vi "TrayROIArr.vi"() -> ()   [LabVIEW 2019]
uses:
  <vilib>/Utility/miscctls.llb/LVRowAndColumnTypeDef.ctl
  <vilib>/Utility/miscctls.llb/LVPointTypeDef.ctl
  <vilib>/vision/Image Controls.llb/IMAQ Image.ctl
  <vilib>/vision/Pattern Matching.llb/IMAQ Pattern Match Advanced Options.ctl
  Auto Inspection Tray Map Name.ctl
  54da9b37-9451-4d09-bda1-2468331c8fce.vi
  3a246969-8a69-47b9-98d6-f50759c243ea.vi
  cc50742a-40e5-4032-86be-5ab09aa8e016.vi
  36dc4686-89ba-4588-a2d3-35b5f35309b2.vi
  d60a80a8-80a4-4e46-9028-f9893c6610f3.vi
  <vilib>/JDP Science/JSONtext/Variant to JSON Text.vi
  <vilib>/JDP Science/JSONtext/JSON text to Variant.vi
  LLB/Commonly VI.lvlib
  <vilib>/vision/NI_Vision_Development_Module.lvlib
  LLB/Commonly VI/Main Glb.vi
panel:
  out "Matches (pixel)":T1(array[cluster]) {"Bounding Box"."y" format="%.2f"; "Bounding Box"."x" format="%.2f"; "Score" format="%.2f"; "Scale" format="%.2f"; "Angle" format="%.2f"; "Position"."y" format="%.2f"; "Position"."x" format="%.2f"}
  in  "ImgCut":bool
  in  "Project":string
  in  "LSCopyFrom":u16(ring) items=["Area1", "Area2"]
  in  "LSXNum":i32 caption="XNum"
  in  "LSYNum":i32 caption="YNum"
  in  "LSXDist":i32 caption="XDist"
  in  "LSYDist":i32 caption="YDist"
  out "LSTotalTrayArea":string[][](table) caption="料盤區塊對應"
  in  "LSAnalysisProject":u16(ring) caption="AnalysisProject" items=["22", "33", "44", "55"]
  in  "AIAnalysisProject":u16(ring) caption="AnalysisProject" items=["22", "33", "44", "55"]
  out "Cell Position":T2
  in  "LSAreaSelect":u16(ring)
  in  "Tab Control":enum32{"LineScan"}(tab)
  in  "Stop Button":bool
  in  "Btn_LSAreaCoordSet":bool
  in  "Save Folder":path
  out "Image":T3(plugin-control)
  in  "Btn_LSAreaDataSet":bool
  out "LS Image":T3(plugin-control)
  in  "Photo":bool
  in  "Btn_LSROITryrun":bool
  in  "Btn_Save":bool
  in  "FolderCut":bool
  in  "Source Folder":path
  in  "定位開啟":bool
  in  "Tab Control 2":enum32{"定位Table", "區域Table"}(tab)
  in  "LSAreaROI 2":i32(listbox) caption="AreaCoordROI"
  in  "LSAreaROI":i32(listbox) caption="AreaROI"
  # "AX     RX個\n\nAY     RY個\n\nN\n\nAY*(N/RX)....."
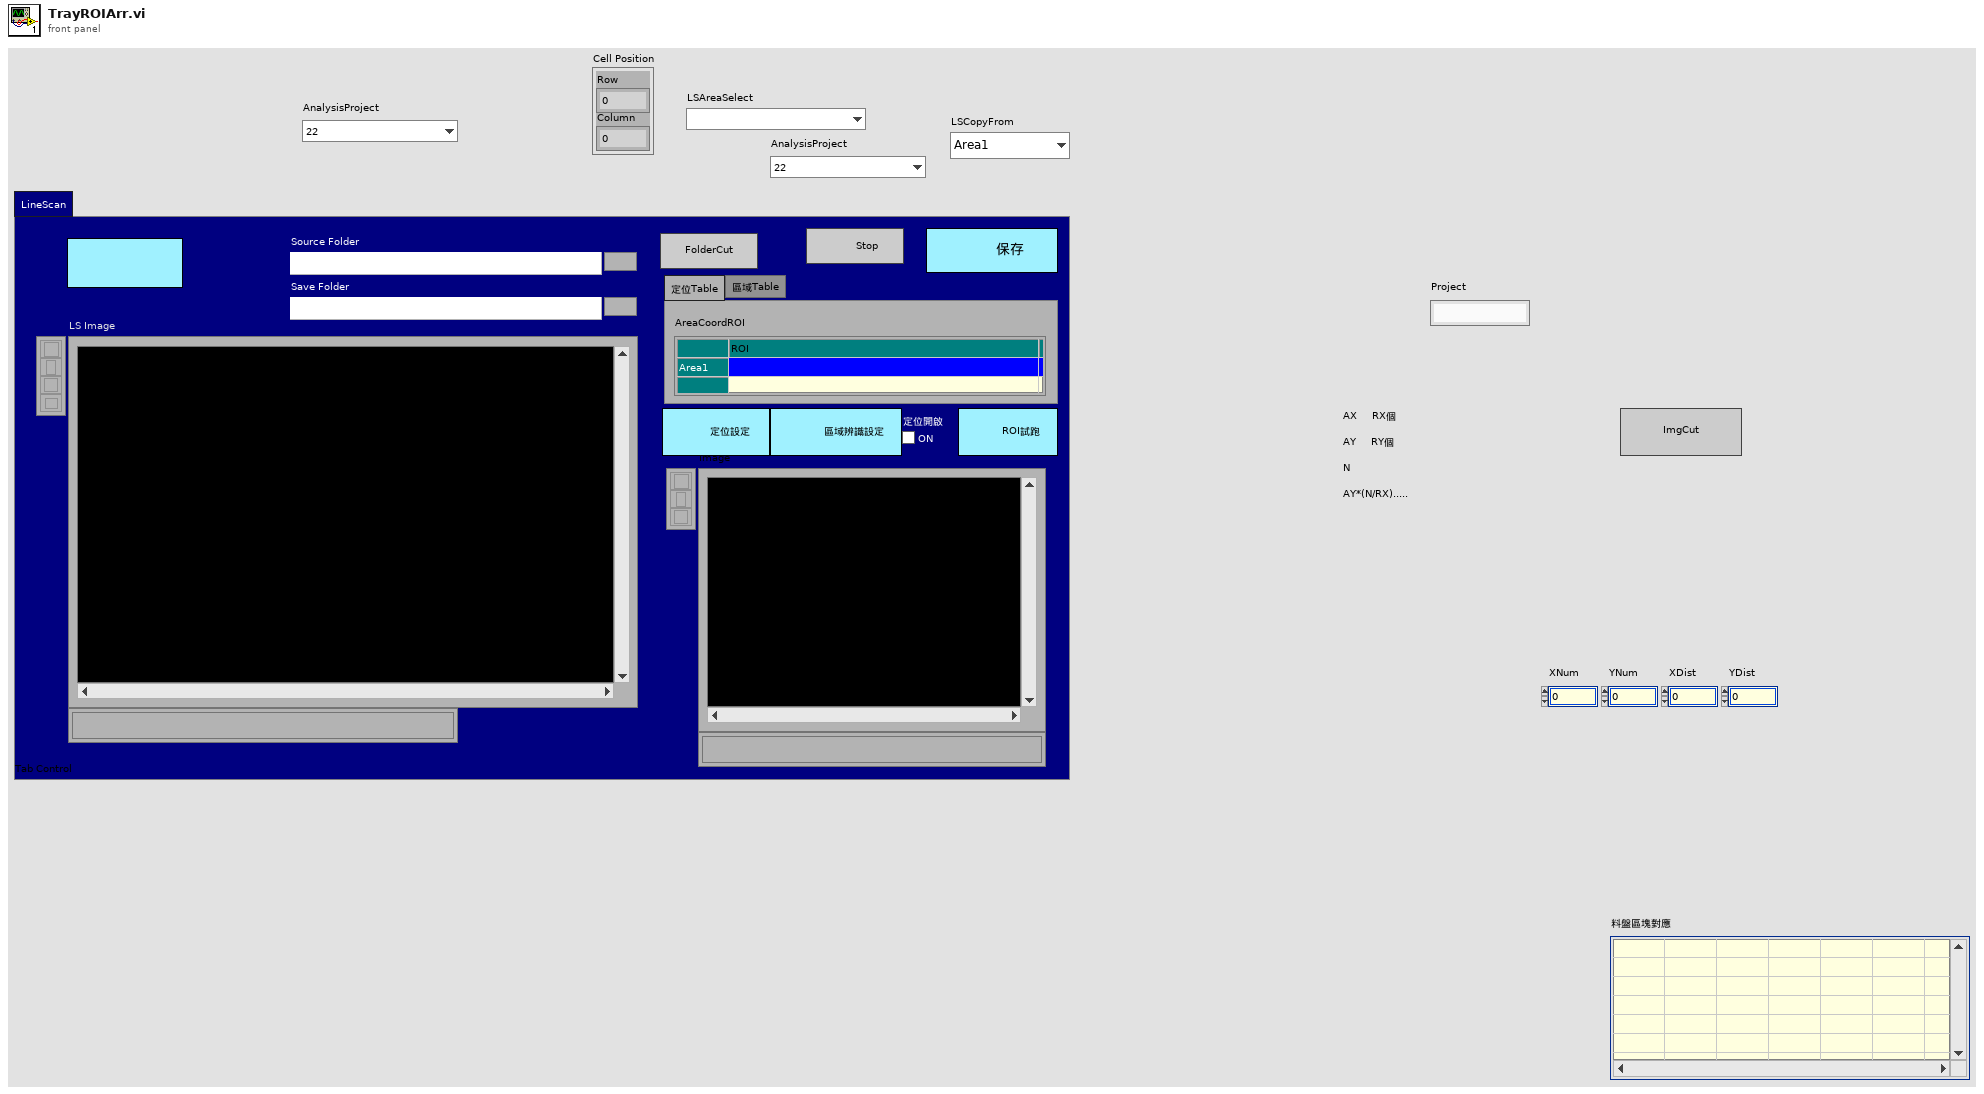
[diagram p1: front panel]
types:
  T1 = cluster{"Position":cluster{"x":sgl, "y":sgl}, "Angle":sgl, "Scale":sgl, "Score":sgl, "Bounding Box":cluster{"x":sgl, "y":sgl}[]}[]
  T2 = typedef "LVRowAndColumnTypeDef.ctl" = cluster{"Row":i32, "Column":i32}
  T3 = typedef "IMAQ Image.ctl" = refnum<image>
  T4 = typedef "LVPointTypeDef.ctl" = cluster{"Horizontal":i16, "Vertical":i16}
  T5 = enum16{"Initial", "Write", "Read", "Save", "Load", "WrteAll"}
  T6 = typedef "IMAQ Pattern Match Advanced Options.ctl" = u16
  T7 = cluster{"Global Rectangle":i32[], "Contours":cluster{"Contour Type":u32, "ROI Type":u32, "Points":i32[]}[]}
  T8 = cluster{"Number of Matches Requested":i32, "Minimum Match Score":sgl, "Angle Ranges":cluster{"Start Angle":sgl, "End Angle":sgl}[]}
  T9 = typedef "Auto Inspection Tray Map Name.ctl" = enum16{"LSTable", "AITable", "LSMap", "AIMap"}
  T10 = typedef "Image Type" = u32
  T11 = typedef "LVPoint32TypeDef.ctl" = cluster{"Horizontal":i32, "Vertical":i32}
  T12 = cluster{"Global Rectangle":i32[], "Contours":cluster{"ID":enum32{"External", "Internal"}, "Type":u32, "Coordinates":i32[]}[]}
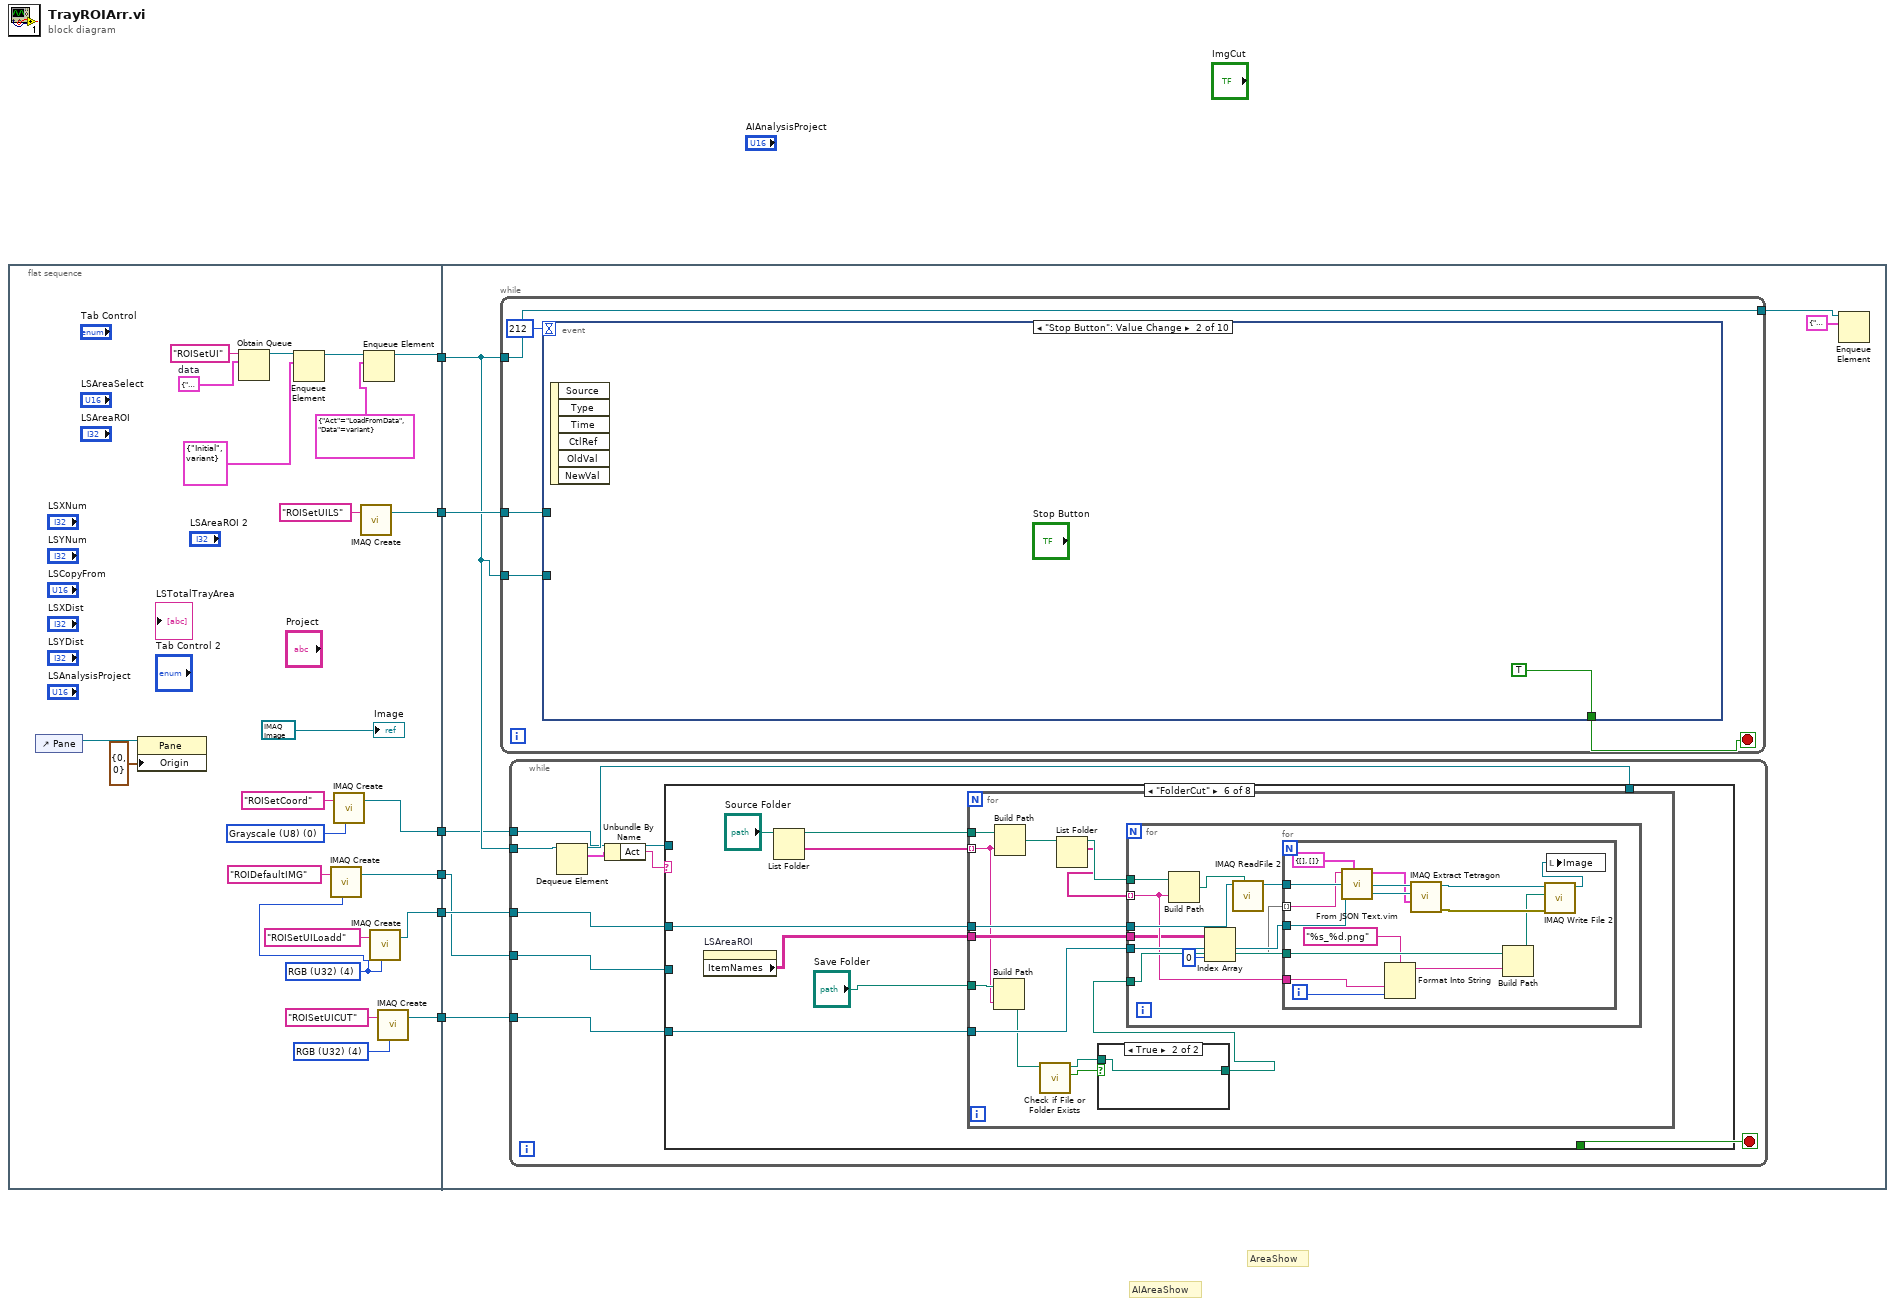
[diagram p0: block diagram]
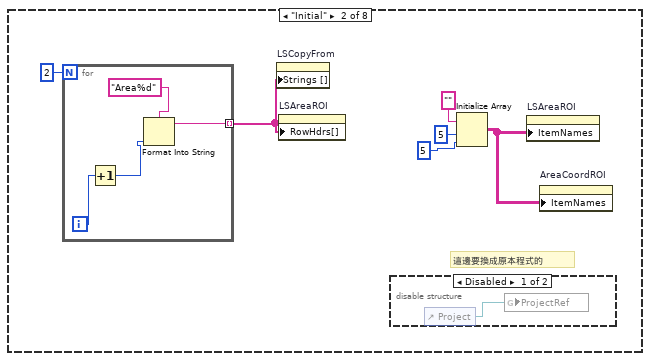
[diagram p3: hidden frame]
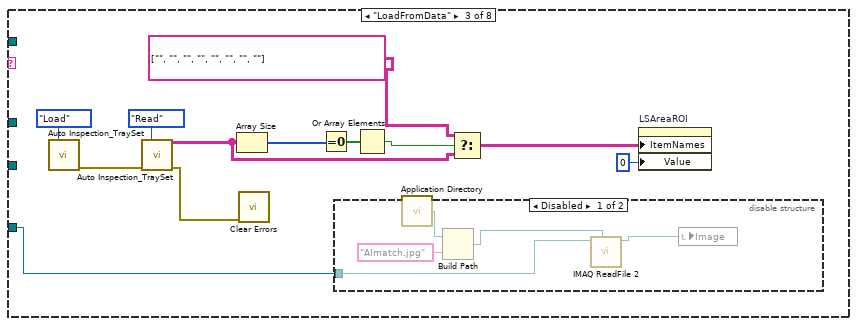
[diagram p5: hidden frame]
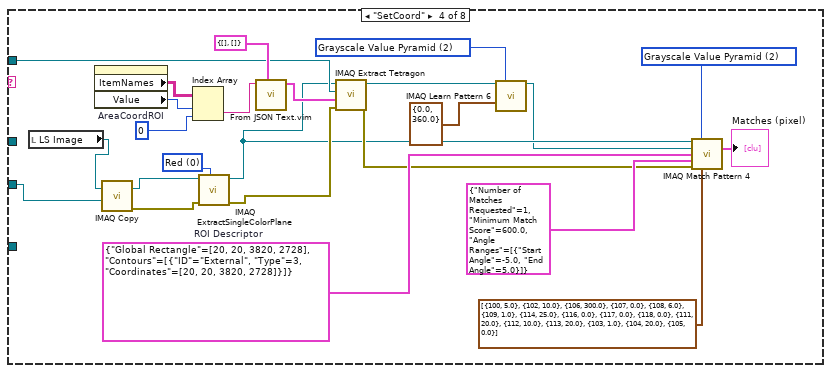
[diagram p7: hidden frame]
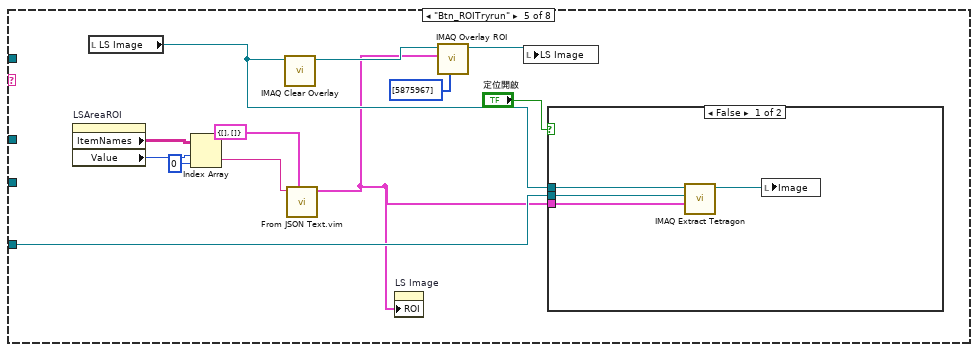
[diagram p8: hidden frame]
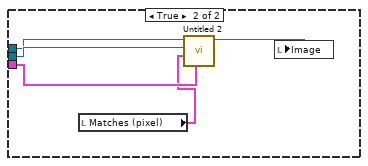
[diagram p9: hidden frame]
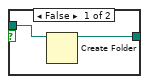
[diagram p10: hidden frame]
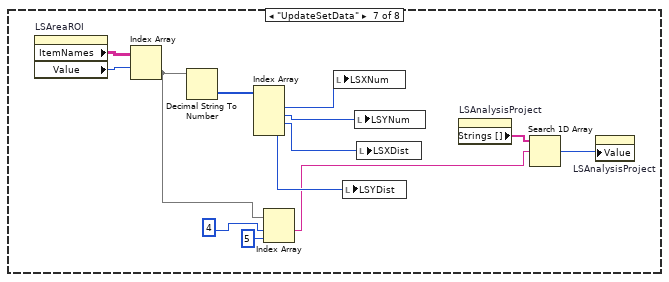
[diagram p11: hidden frame]
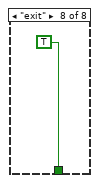
[diagram p12: hidden frame]
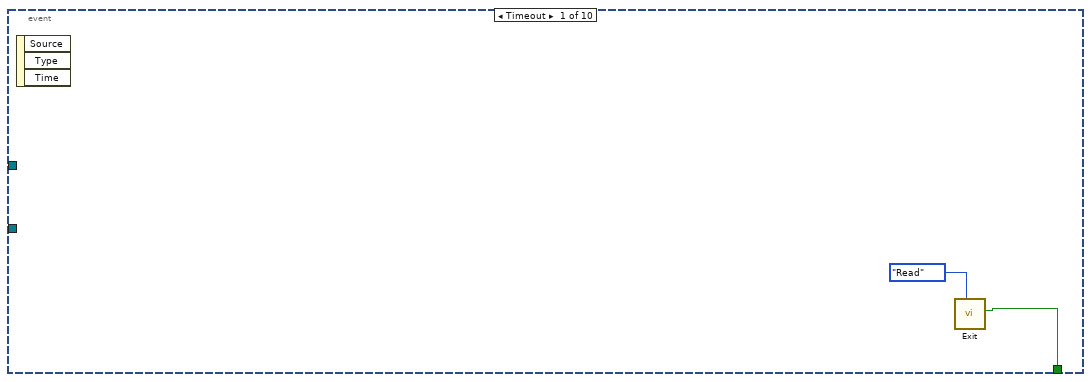
[diagram p13: hidden frame]
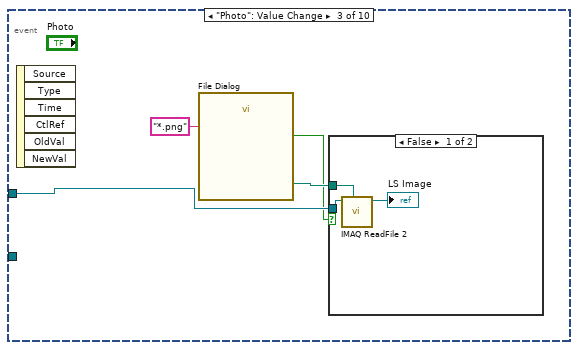
[diagram p14: hidden frame]
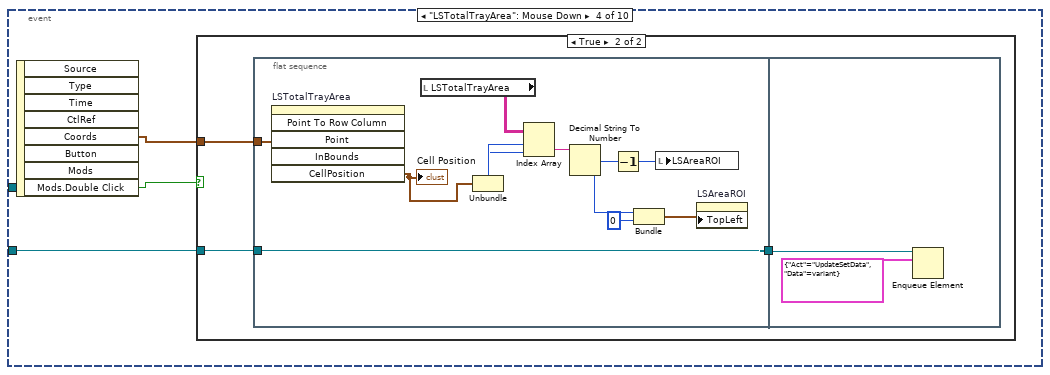
[diagram p16: hidden frame]
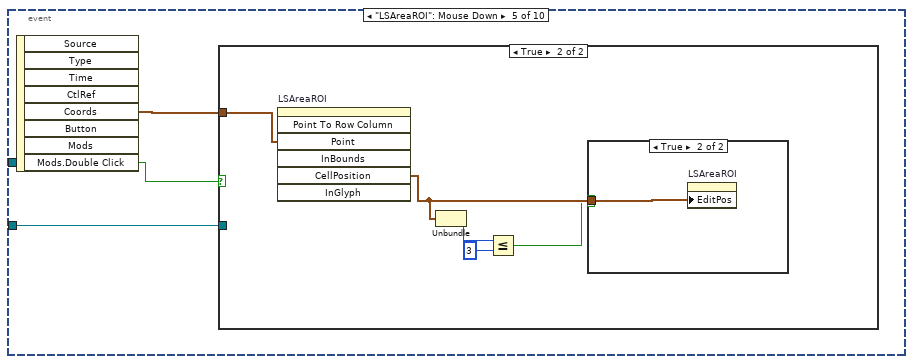
[diagram p18: hidden frame]
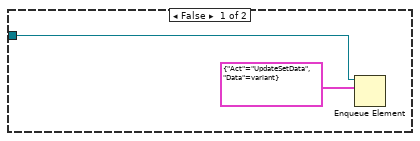
[diagram p19: hidden frame]
diagram:
  # "AreaShow"
  # "AIAreaShow"
  n1 = flat-sequence {
    tunnel: [w21] -> w6
    tunnel: [w24] -> w5
    tunnel: [w16] -> w4
    tunnel: [w14] -> w3
    tunnel: [w12] -> w2
    tunnel: [w10] -> w1
    tunnel: w6 -> [w34]
    tunnel: w5 -> [w35]
    tunnel: w4 -> [w33]
    tunnel: w3 -> [w32]
    tunnel: w2 -> [w31]
    tunnel: w1 -> [w30]
    frame #0 {
      w8 = T10 0 items=["Grayscale (U8)", "Grayscale (I16)", "Grayscale (SGL)", "Complex (CSG)", "RGB (U32)", "HSL (U32)", "RGB (U64)", "Grayscale (U16)"] ("Image Type")
      w9 = T10 4 items=["Grayscale (U8)", "Grayscale (I16)", "Grayscale (SGL)", "Complex (CSG)", "RGB (U32)", "HSL (U32)", "RGB (U64)", "Grayscale (U16)"] ("Image Type")
      w17 = T10 4 items=["Grayscale (U8)", "Grayscale (I16)", "Grayscale (SGL)", "Complex (CSG)", "RGB (U32)", "HSL (U32)", "RGB (U64)", "Grayscale (U16)"] ("Image Type")
      w28 = cluster{"Act":string, "Data":variant} {"Act"="", "Data"=variant}  # data
      n2 = control-ref of="Pane"() -> (w23:refnum<vi>)
      n3 = property class="Pane"(reference=w23, "Origin"=T4 {"Horizontal"=0, "Vertical"=0}) -> ()  [unwired: 1 in, 2 out]
      n4 = Obtain Queue(name (unnamed)="ROISetUI", element data type=w28) -> (queue out=w27:refnum<queue>)  [unwired: 3 in, 2 out]
      n5 = Enqueue Element(queue=w27, element=cluster{"Act":string, "Data":variant} {"Act"="Initial", "Data"=variant}) -> (queue out=w20:refnum<queue>)  [unwired: 2 in, 2 out]
      n6 = call "IMAQ Create"("Image Name"="ROIDefaultIMG", "Image Type"=w9) -> ("New Image"=w10:T3)  [unwired: 3 in, 1 out]
      n7 = call "IMAQ Create"("Image Name"="ROISetCoord", "Image Type"=w8) -> ("New Image"=w12:T3)  [unwired: 3 in, 1 out]
      n8 = call "IMAQ Create"("Image Name"="ROISetUILS") -> ("New Image"=w24:T3)  [unwired: 4 in, 1 out]
      n9 = Enqueue Element(queue=w20, element=cluster{"Act":string, "Data":variant} {"Act"="LoadFromData", "Data"=variant}) -> (queue out=w21:refnum<queue>)  [unwired: 2 in, 2 out]
      n10 = call "IMAQ Create"("Image Name"="ROISetUILoadd", "Image Type"=w9) -> ("New Image"=w14:T3)  [unwired: 3 in, 1 out]
      n11 = call "IMAQ Create"("Image Name"="ROISetUICUT", "Image Type"=w17) -> ("New Image"=w16:T3)  [unwired: 3 in, 1 out]
      "Image" <- T3 refnum ("Image")
    }
    frame #1 {
      n12 = while {
        tunnel: w34 -> [w185]
        tunnel: [w185] -> w37
        tunnel: w35 -> [w182]
        tunnel: w34 -> [w181]
        stop <- w183 stop-if-true
        n13 = event shown="[1] \"Stop Button\": Value Change" {
          selector: _ -> [_ _ _ _ _ _ _ _ _ _]
          dyn-events: _ -> [_ _ _ _ _ _ _ _ _ _]
          timeout: 212 -> [_ _ _ _ _ _ _ _ _ _]
          tunnel: [w186 TRUE _ _ _ _ _ _ _ _] -> w183
          tunnel: w182 -> [_ _ w190 _ _ _ _ _ _ _]
          tunnel: w181 -> [_ _ _ w196 w217 _ w238 w248 _ w259]
          event Timeout {
            n14 = event-data() -> ()  [unwired: 1 in, 3 out]
            n15 = call "Exit.vi"("Enum"=enum16{"Initial", "Read", "Write"}."Read") -> ("ExitOut"=w186:bool)  [unwired: 10 in]
          }
          event "Stop Button": Value Change {
            n16 = event-data() -> ()  [unwired: 1 in, 6 out]
          }
          event "Photo": Value Change {
            n17 = event-data() -> ()  [unwired: 1 in, 6 out]
            n18 = call "File Dialog"("pattern (all files)"="*.png") -> ("selected path"=w191:path, "cancelled"=w189:bool)  [unwired: 11 in, 2 out]
            n19 = case shown="False" w189 {
              tunnel: w191 -> [w195 _]
              tunnel: w190 -> [w194 _]
              frame False {
                n20 = call "IMAQ ReadFile 2"("File Path"=w195, "Image"=w194) -> ("Image Out"=→"LS Image":T3)  [unwired: 5 in, 4 out]
              }
              frame True {
              }
            }
          }
          event "LSTotalTrayArea": Mouse Down {
            n21 = event-data() -> ("Coords"=w197:T11, "Mods.Double Click"=w198:bool)  [unwired: 1 in, 6 out]
            n22 = case shown="True" w198 {
              tunnel: w197 -> [_ w201]
              tunnel: w196 -> [_ w199]
              frame False {
              }
              frame True {
                n23 = flat-sequence {
                  tunnel: w201 -> [w212]
                  tunnel: [w202] -> w200
                  tunnel: w199 -> [w202]
                  tunnel: w200 -> [w214]
                  frame #0 {
                    n24 = invoke on="LSTotalTrayArea" class="Tbl (strict)" method="Point To Row Column"("Point"=w212) -> ("CellPosition"=w210:T2)  [unwired: 5 in, 5 out]
                    "Cell Position" <- w210
                    n25 = local read "LSTotalTrayArea"() -> (w211:string[][])
                    n26 = Unbundle(w210) -> ("Row"=w209:i32, "Column"=w208:i32)
                    n27 = Index Array(array=w211, index (row)=w209, index (col)=w208) -> (element=w207:string)
                    n28 = Decimal String To Number(string=w207) -> (number=w206:i32)  [unwired: 2 in, 1 out]
                    n29 = Decrement(x=w206) -> (x-1=w204:i32)
                    n30 = Bundle(w204, 0) -> (w205:cluster{i32, i32})  [unwired: 1 in]
                    n31 = local write "LSAreaROI"(w204) -> ()
                    n32 = property on="LSAreaROI" class="MCListbox (strict)"("TopLeft"=w205) -> ()  [unwired: 2 in, 2 out]
                  }
                  frame #1 {
                    n33 = Enqueue Element(queue=w214, element=cluster{"Act":string, "Data":variant} {"Act"="UpdateSetData", "Data"=variant}) -> ()  [unwired: 2 in, 3 out]
                  }
                }
              }
            }
          }
          event "LSAreaROI": Mouse Down {
            n34 = event-data() -> ("Coords"=w215:T11, "Mods.Double Click"=w216:bool)  [unwired: 1 in, 6 out]
            n35 = case shown="True" w216 {
              tunnel: w217 -> [w219 _]
              tunnel: w215 -> [_ w224]
              frame False {
                n36 = Enqueue Element(queue=w219, element=cluster{"Act":string, "Data":variant} {"Act"="UpdateSetData", "Data"=variant}) -> ()  [unwired: 2 in, 3 out]
              }
              frame True {
                n37 = invoke on="LSAreaROI" class="MCListbox (strict)" method="Point To Row Column"("Point"=w224) -> ("CellPosition"=w223:T2)  [unwired: 6 in, 6 out]
                n38 = Unbundle(w223) -> ("Column"=w222:i32)  [unwired: 1 out]
                n39 = Less Or Equal?(x=w222, y=3) -> (x <= y?=w220:bool)
                n40 = case shown="True" w220 {
                  tunnel: w223 -> [_ w225]
                  frame False {
                  }
                  frame True {
                    n41 = property on="LSAreaROI" class="MCListbox (strict)"("EditPos"=w225) -> ()  [unwired: 2 in, 2 out]
                  }
                }
              }
            }
          }
          event "Btn_LSAreaDataSet": Value Change {
            n42 = event-data() -> ()  [unwired: 1 in, 6 out]
            n43 = property on="LSAreaROI" class="MCListbox (strict)"() -> ("ItemNames"=w231:string[][], "Value"=w228:i32)  [unwired: 2 in, 2 out]
            n44 = property on="LS Image" class="ImageControl"() -> ("ROI"=w227:T7)  [unwired: 2 in, 2 out]
            n45 = call "To JSON Text.vim"("Anything"=w227) -> ("<JSON>"=w226:string)  [unwired: 9 in, 1 out]
            n46 = Build Array(w226) -> (w229:string[])
            n47 = Replace Array Subset(array=w231, new element=w229, index (row)=w228) -> (w230:string[][])  [unwired: 1 in]
            n48 = property on="LSAreaROI" class="MCListbox (strict)"("ItemNames"=w230) -> ()  [unwired: 2 in, 2 out]
          }
          event "Btn_LSAreaCoordSet": Value Change {
            n49 = event-data() -> ()  [unwired: 1 in, 6 out]
            n50 = property on="AreaCoordROI" class="MCListbox (strict)"() -> ("ItemNames"=w246:string[][], "Value"=w245:i32)  [unwired: 2 in, 2 out]
            n51 = property on="LS Image" class="ImageControl"() -> ("ROI"=w241:T7)  [unwired: 2 in, 2 out]
            n52 = call "To JSON Text.vim"("Anything"=w241) -> ("<JSON>"=w244:string)  [unwired: 9 in, 1 out]
            n53 = Build Array(w244) -> (w243:string[])
            n54 = local read "LS Image"() -> (w240:T3)
            n55 = Replace Array Subset(array=w246, new element=w243, index (row)=w245) -> (w242:string[][])  [unwired: 1 in]
            n56 = call-poly "IMAQ Extract Tetragon"("ROI Descriptor"=w241, "Image Dst"="ROISetUICUT" ("Image Name"), "Image Src"=w240) -> ("Image Dst Out"=w235:T3)  [unwired: 7 in, 1 out]
            n57 = call <vilib>:"Application Directory.vi"() -> ("Application Directory"=w234:path)
            n58 = property on="AreaCoordROI" class="MCListbox (strict)"("ItemNames"=w242) -> (error out=w236:errorcluster)  [unwired: 2 in, 1 out]
            n59 = Build Path(base path=w234, name or relative path="AImatch.jpg") -> (appended path=w233:path)
            n60 = local write "Image"(w235) -> ()
            n61 = call-poly "IMAQ Write File 2"("File Path"=w233, "Image"=w235) -> ()  [unwired: 8 in, 2 out]
            n62 = Enqueue Element(queue=w238, element=cluster{"Act":string, "Data":variant} {"Act"="SetCoord", "Data"=variant}, error in (no error)=w236) -> ()  [unwired: 1 in, 3 out]
          }
          event "Btn_LSROITryrun": Value Change {
            n63 = event-data() -> ()  [unwired: 1 in, 6 out]
            n64 = Enqueue Element(queue=w248, element=cluster{"Act":string, "Data":variant} {"Act"="Btn_ROITryrun", "Data"=variant}) -> ()  [unwired: 2 in, 3 out]
          }
          event "Btn_Save": Value Change {
            n65 = event-data() -> ()  [unwired: 1 in, 6 out]
            n66 = property on="LSAreaROI 2" class="MCListbox (strict)" props=["ItemNames"]() -> ()  [unwired: 2 in, 3 out]
            n67 = property on="LSAreaROI" class="MCListbox (strict)"() -> ("ItemNames"=w256:string[][])  [unwired: 2 in, 2 out]
            n68 = call "Auto Inspection_TraySet.vi"("TableIn"=w256, "Action"=T5."WrteAll", "Name"=Auto_Inspection_Tray_Map_Name."LSTable") -> ("error out"=w250:errorcluster)  [unwired: 7 in, 5 out]
            n69 = property on="LSTotalTrayArea" class="Tbl (strict)"() -> ("Value"=w252:string[][])  [unwired: 2 in, 2 out]
            n70 = call "Auto Inspection_TraySet.vi"("TableIn"=w252, "Action"=T5."WrteAll", "error in"=w250, "Name"=Auto_Inspection_Tray_Map_Name."LSMap") -> ("error out"=w249:errorcluster)  [unwired: 6 in, 5 out]
            n71 = call "Auto Inspection_TraySet.vi"("Action"=T5."Save", "error in"=w249) -> ()  [unwired: 8 in, 6 out]
          }
          event "FolderCut": Value Change {
            n72 = event-data() -> ()  [unwired: 1 in, 3 out]
            n73 = Enqueue Element(queue=w259, element=cluster{"Act":string, "Data":variant} {"Act"="FolderCut", "Data"=variant}) -> ()  [unwired: 2 in, 3 out]
          }
        }
      }
      n74 = while {
        tunnel: w34 -> [w46]
        tunnel: w33 -> [w41]
        tunnel: w32 -> [w40]
        tunnel: w31 -> [w39]
        tunnel: w30 -> [w38]
        stop <- w43 stop-if-true
        n75 = Dequeue Element(queue=w46) -> (queue out=w42:refnum<queue>, element=w45:cluster{"Act":string, "Data":variant})  [unwired: 2 in, 2 out]
        n76 = Unbundle By Name(w45) -> ("Act"=w44:string)
        n77 = case shown="\"FolderCut\"" w44 {
          tunnel: [_ _ _ _ _ _ _ TRUE] -> w43
          tunnel: w42 -> [_ _ _ _ _ _ _ _]
          tunnel: w41 -> [_ _ w58 _ w102 w123 _ _]
          tunnel: w40 -> [_ _ _ _ _ w122 _ _]
          tunnel: w39 -> [_ _ _ w91 _ _ _ _]
          tunnel: w38 -> [_ _ _ w85 _ _ _ _]
          frame "False", Default {
          }
          frame "Initial" {
            # "這邊要換成原本程式的"
            n78 = for {
              N: 2 -> [_]
              tunnel: [w56] -> w51 mode=indexing
              i -> [w55]
              n79 = Increment(x=w55) -> (x+1=w54:i32)
              n80 = Format Into String(format string="Area%d", w54) -> (resulting string=w56:string)  [unwired: 2 in, 1 out]
            }
            n81 = property on="LSCopyFrom" class="Ring (strict)"("Strings []"=w51) -> ()  [unwired: 2 in, 2 out]
            n82 = property on="LSAreaROI" class="MCListbox (strict)"("RowHdrs[]"=w51) -> ()  [unwired: 2 in, 2 out]
            n83 = disable-structure shown="Disabled" {
              frame Disabled {
                n84 = control-ref of="Project"() -> (w53:refnum<vi>)
                n85 = global write "Main Glb.vi" "ProjectRef"(w53) -> ()
              }
              frame Enabled {
              }
            }
            n86 = Initialize Array("", 5 ("dimension size"), 5 ("dimension size")) -> (w47:string[][])
            n87 = property on="LSAreaROI" class="MCListbox (strict)"("ItemNames"=w47) -> ()  [unwired: 2 in, 2 out]
            n88 = property on="AreaCoordROI" class="MCListbox (strict)"("ItemNames"=w47) -> ()  [unwired: 2 in, 2 out]
          }
          frame "LoadFromData" {
            n89 = call "Auto Inspection_TraySet.vi"("Action"=T5."Load") -> ("error out"=w67:errorcluster)  [unwired: 9 in, 5 out]
            n90 = call "Auto Inspection_TraySet.vi"("Action"=T5."Read", "error in"=w67) -> ("LSTableOut"=w62:string[][], "error out"=w59:errorcluster)  [unwired: 8 in, 4 out]
            n91 = Array Size(array=w62) -> (size(s)=w65:i32[])
            n92 = call <vilib>:"Clear Errors.vi"("error in (no error)"=w59) -> ()  [unwired: 5 in, 2 out]
            n93 = Equal To 0?(x=w65) -> (x = 0?=w64:bool[])
            n94 = disable-structure shown="Disabled" {
              disable-tunnel: w58 -> [w72 _]
              frame Disabled {
                n95 = call <vilib>:"Application Directory.vi"() -> ("Application Directory"=w73:path)
                n96 = Build Path(base path=w73, name or relative path="AImatch.jpg") -> (appended path=w71:path)
                n97 = call "IMAQ ReadFile 2"("File Path"=w71, "Image"=w72) -> ("Image Out"=w70:T3)  [unwired: 5 in, 4 out]
                n98 = local write "Image"(w70) -> ()
              }
              frame Enabled {
              }
            }
            n99 = Or Array Elements(Boolean array=w64) -> (logical OR=w63:bool)
            n100 = Select(t=string[][] [["", "", "", ""], ["", "", "", ""]], s=w63, f=w62) -> (s? t:f=w61:string[][])
            n101 = property on="LSAreaROI" class="MCListbox (strict)"("ItemNames"=w61, "Value"=0 ("LSAreaROI")) -> ()  [unwired: 2 in, 2 out]
          }
          frame "SetCoord" {
            w79 = 2 items=["All", "Low Discrepancy Sampling", "Grayscale Value Pyramid", "Gradients Pyramid"] ("Algorithm")
            w84 = T12 {"Global Rectangle"=[20, 20, 3820, 2728], "Contours"=[{"ID"=enum."External", "Type"=3, "Coordinates"=[20, 20, 3820, 2728]}]}  # ROI Descriptor
            w89 = 0 items=["Red", "Green", "Blue", "Hue", "Saturation", "Luminance", "Value", "Intensity"] ("Color Plane")
            w97 = 2 items=["All", "Low Discrepancy Sampling", "Grayscale Value Pyramid", "Gradients Pyramid"] ("Algorithm")
            n102 = local read "LS Image"() -> (w86:T3)
            n103 = property on="AreaCoordROI" class="MCListbox (strict)"() -> ("ItemNames"=w98:string[][], "Value"=w94:i32)  [unwired: 2 in, 2 out]
            n104 = call "IMAQ Copy"("Image Dst"=w85, "Image Src"=w86) -> ("error out"=w87:errorcluster, "Image Dst Out"=w88:T3)  [unwired: 4 in]
            n105 = Index Array(array=w98, index (row)=w94, index (col)=0 ("index (row)")) -> (element=w92:string)
            n106 = call "IMAQ ExtractSingleColorPlane"("Color Plane"=w89, "error in (no error)"=w87, "Image Src"=w88) -> ("error out"=w82:errorcluster, "Image Dst Out"=w80:T3)  [unwired: 1 in, 6 out]
            n107 = call "From JSON Text.vim"("Data Type and Default Value"=T7 {"Global Rectangle"=[], "Contours"=[]} ("ROI"), "JSON"=w92) -> ("Data out"=w90:T7)  [unwired: 8 in, 1 out]
            n108 = call-poly "IMAQ Extract Tetragon"("error in (no error)"=w82, "ROI Descriptor"=w90, "Image Dst"=w91, "Image Src"=w80) -> ("error out"=w81:errorcluster, "Image Dst Out"=w78:T3)  [unwired: 6 in]
            n109 = call "IMAQ Learn Pattern 6"("Image"=w78, "Algorithm"=w79, "Angle Range"=cluster{"Start Angle":sgl, "End Angle":sgl} {"Start Angle"=0.0, "End Angle"=360.0}) -> ("Template Image Out"=w76:T3)  [unwired: 10 in, 2 out]
            n110 = call "IMAQ Match Pattern 4"("Image"=w80, "Algorithm"=w97, "Template Image"=w76, "ROI Descriptor"=w84, "Parameters"=T8 {"Number of Matches Requested"=1, "Minimum Match Score"=600.0, "Angle Ranges"=[{"Start Angle"=-5.0, "End Angle"=5.0}]}, "error in (no error)"=w81, "Advanced Options"=cluster{"Item":T6, "Value":dbl}[] [{"Item"=100, "Value"=5.0}, {"Item"=102, "Value"=10.0}, {"Item"=106, "Value"=300.0}, {"Item"=107, "Value"=0.0}, {"Item"=108, "Value"=6.0}, {"Item"=109, "Value"=1.0}, {"Item"=114, "Value"=25.0}, {"Item"=116, "Value"=0.0}, {"Item"=117, "Value"=0.0}, {"Item"=118, "Value"=0.0}, {"Item"=111, "Value"=20.0}, {"Item"=112, "Value"=10.0}, {"Item"=113, "Value"=20.0}, {"Item"=103, "Value"=1.0}, {"Item"=104, "Value"=20.0}, {"Item"=105, "Value"=0.0}]) -> ("Matches (pixel)"=→"Matches (pixel)":T1)  [unwired: 4 in, 4 out]
          }
          frame "Btn_ROITryrun" {
            n111 = property on="LSAreaROI" class="MCListbox (strict)"() -> ("ItemNames"=w107:string[][], "Value"=w106:i32)  [unwired: 2 in, 2 out]
            n112 = local read "LS Image"() -> (w101:T3)
            n113 = Index Array(array=w107, index (row)=w106, index (col)=0 ("disabled index (col)")) -> (element=w104:string)
            n114 = call "IMAQ Clear Overlay"("Image"=w101) -> ("Image Out"=w110:T3)  [unwired: 9 in, 1 out]
            n115 = call "From JSON Text.vim"("Data Type and Default Value"=T7 {"Global Rectangle"=[], "Contours"=[]} ("ROI"), "JSON"=w104) -> ("Data out"=w100:T7)  [unwired: 8 in, 1 out]
            n116 = property on="LS Image" class="ImageControl"("ROI"=w100) -> ()  [unwired: 2 in, 2 out]
            n117 = call "IMAQ Overlay ROI"("Colors (Green)"=u32[] [5875967], "ROI Descriptor"=w100, "Image"=w110) -> ("Image Out"=w109:T3)  [unwired: 7 in, 1 out]
            n118 = local write "LS Image"(w109) -> ()
            n119 = case shown="False" "定位開啟" {
              tunnel: w102 -> [w114 w117]
              tunnel: w101 -> [w113 w116]
              tunnel: w100 -> [w112 w118]
              frame False {
                n120 = call-poly "IMAQ Extract Tetragon"("ROI Descriptor"=w112, "Image Dst"=w114, "Image Src"=w113) -> ("Image Dst Out"=w111:T3)  [unwired: 7 in, 1 out]
                n121 = local write "Image"(w111) -> ()
              }
              frame True {
                n122 = local read "Matches (pixel)"() -> (w115:T1)
                n123 = call "Untitled 2.vi"("ROI Descriptor"=w118, "Matches (pixel)"=w115, "Image Dst"=w117, "Image in"=w116) -> ("Image Dst Out"=w119:T3)  [unwired: 7 in]
                n124 = local write "Image"(w119) -> ()
              }
            }
          }
          frame "FolderCut" {
            n125 = property on="LSAreaROI" class="MCListbox (strict)"() -> ("ItemNames"=w121:string[][])  [unwired: 2 in, 2 out]
            n126 = List Folder(path="Source Folder") -> (path out=w125:path, folder names=w124:string[])  [unwired: 3 in, 2 out]
            n127 = for {
              tunnel: w125 -> [w139]
              tunnel: w124 -> [w131] mode=indexing
              tunnel: w123 -> [w135]
              tunnel: w122 -> [w134]
              tunnel: w121 -> [w133]
              tunnel: "Save Folder" -> [w132]
              n128 = Build Path(base path=w132, name or relative path=w131) -> (appended path=w130:path)
              n129 = Build Path(base path=w139, name or relative path=w131) -> (appended path=w138:path)
              n130 = call <vilib>:"Check if File or Folder Exists.vi"("path"=w130) -> ("file or folder exists?"=w129:bool, "dup path"=w128:path)  [unwired: 8 in, 1 out]
              n131 = List Folder(path=w138) -> (path out=w137:path, filenames=w136:string[])  [unwired: 3 in, 2 out]
              n132 = case shown="True" w129 {
                tunnel: w128 -> [w141 w142]
                tunnel: [w140 w142] -> w127
                frame False {
                  n133 = Create Folder(path (use dialog)=w141) -> (created path=w140:path)  [unwired: 2 in, 2 out]
                }
                frame True {
                }
              }
              n134 = for {
                tunnel: w137 -> [w152]
                tunnel: w136 -> [w146] mode=indexing
                tunnel: w135 -> [w148]
                tunnel: w134 -> [w150]
                tunnel: w133 -> [w145]
                tunnel: w127 -> [w147]
                n135 = Build Path(base path=w152, name or relative path=w146) -> (appended path=w151:path)
                n136 = Index Array(array=w145, index (col)=0 ("disabled index (col)")) -> (element=w143:string[])  [unwired: 1 in]
                n137 = call "IMAQ ReadFile 2"("File Path"=w151, "Image"=w150) -> ("Image Out"=w149:T3)  [unwired: 5 in, 4 out]
                n138 = for {
                  tunnel: w149 -> [w166]
                  tunnel: w148 -> [w165]
                  tunnel: w143 -> [w164] mode=indexing
                  tunnel: w147 -> [w159]
                  tunnel: w146 -> [w157]
                  i -> [w156]
                  n139 = call "From JSON Text.vim"("Data Type and Default Value"=T7 {"Global Rectangle"=[], "Contours"=[]} ("ROI"), "JSON"=w164) -> ("Data out"=w162:T7)  [unwired: 8 in, 1 out]
                  n140 = Format Into String(format string="%s_%d.png", w157, w156) -> (resulting string=w155:string)  [unwired: 2 in, 1 out]
                  n141 = call-poly "IMAQ Extract Tetragon"("ROI Descriptor"=w162, "Image Dst"=w165, "Image Src"=w166) -> ("error out"=w161:errorcluster, "Image Dst Out"=w160:T3)  [unwired: 7 in]
                  n142 = Build Path(base path=w159, name or relative path=w155) -> (appended path=w154:path)
                  n143 = call-poly "IMAQ Write File 2"("error in (no error)"=w161, "File Path"=w154, "Image"=w160) -> ("Image Out (duplicate)"=w153:T3)  [unwired: 7 in, 1 out]
                  n144 = local write "Image"(w153) -> ()
                }
              }
            }
          }
          frame "UpdateSetData" {
            n145 = property on="LSAreaROI" class="MCListbox (strict)"() -> ("ItemNames"=w179:string[][], "Value"=w178:i32)  [unwired: 2 in, 2 out]
            n146 = Index Array(array=w179, index (row)=w178) -> (element=w172:string[])  [unwired: 1 in]
            n147 = Decimal String To Number(string=w172) -> (number=w177:i32[])  [unwired: 2 in, 1 out]
            n148 = Index Array(array=w177) -> (element #1=w176:i32, element #2=w175:i32, element #3=w174:i32, element #4=w173:i32)  [unwired: 4 in]
            n149 = Index Array(array=w172, index #1=4 ("index"), index #2=5 ("index")) -> (element #1=w168:string)  [unwired: 1 out]
            n150 = local write "LSXNum"(w176) -> ()
            n151 = local write "LSYDist"(w173) -> ()
            n152 = local write "LSYNum"(w175) -> ()
            n153 = local write "LSXDist"(w174) -> ()
            n154 = property on="LSAnalysisProject" class="Ring (strict)"() -> ("Strings []"=w169:string[])  [unwired: 2 in, 2 out]
            n155 = Search 1D Array(1D array=w169, element=w168) -> (index of element=w167:i32)  [unwired: 1 in]
            n156 = property on="LSAnalysisProject" class="Ring (strict)"("Value"=w167) -> ()  [unwired: 2 in, 2 out]
          }
          frame "exit" {
          }
        }
      }
      n157 = Enqueue Element(queue=w37, element=cluster{"Act":string, "Data":variant} {"Act"="exit", "Data"=variant}) -> ()  [unwired: 2 in, 3 out]
    }
  }
